vi "Raster_2DOutput_wCounter_82_EXP_ODMR pulsing.vi"(2 "Save File path":path, 3 "Save?":bool=TRUE, 6 "error in":errorcluster, 7 "Update Rate (Hz)":dbl=100.0, 8 "Y Parameters":T1={"Number of Y Steps"=200, "Max Y (V)"=1.0, "Min Y (V)"=-1.0}, 9 "X Parameters":T2={"Number of X Steps"=200, "Max X (V)"=1.0, "Min X (V)"=-1.0}) -> (0 "error out":errorcluster, 1 "Intensity Graph":dbl[][](graph))   [LabVIEW 2012]
uses:
  <vilib>/DAQmx/write.llb/DAQmx Write (Analog 2D DBL NChan NSamp).vi
  <vilib>/DAQmx/read.llb/DAQmx Read (Counter 1D U32 1Chan NSamp).vi
  <vilib>/DAQmx/create/channels.llb/DAQmx Create Channel (CI-Count Edges).vi
  <vilib>/DAQmx/create/channels.llb/DAQmx Create Channel (AO-Voltage-Basic).vi
  <vilib>/DAQmx/configure/timing.llb/DAQmx Timing (Sample Clock).vi
  <vilib>/DAQmx/miscellaneous.llb/DAQmx Fill In Error Info.vi
  <resource>/objmgr/daqmx.rc
panel:
  out "Intensity Graph 3":dbl[][](graph)
  out "Intensity Graph 2":dbl[][](graph)
  out "TotalSampPerChanAcquired 2":dbl=5601.0
  out "TotalSampPerChanAcquired":dbl=5601.0
  out "Output:":dbl[][](graph)
  in  "stop":bool
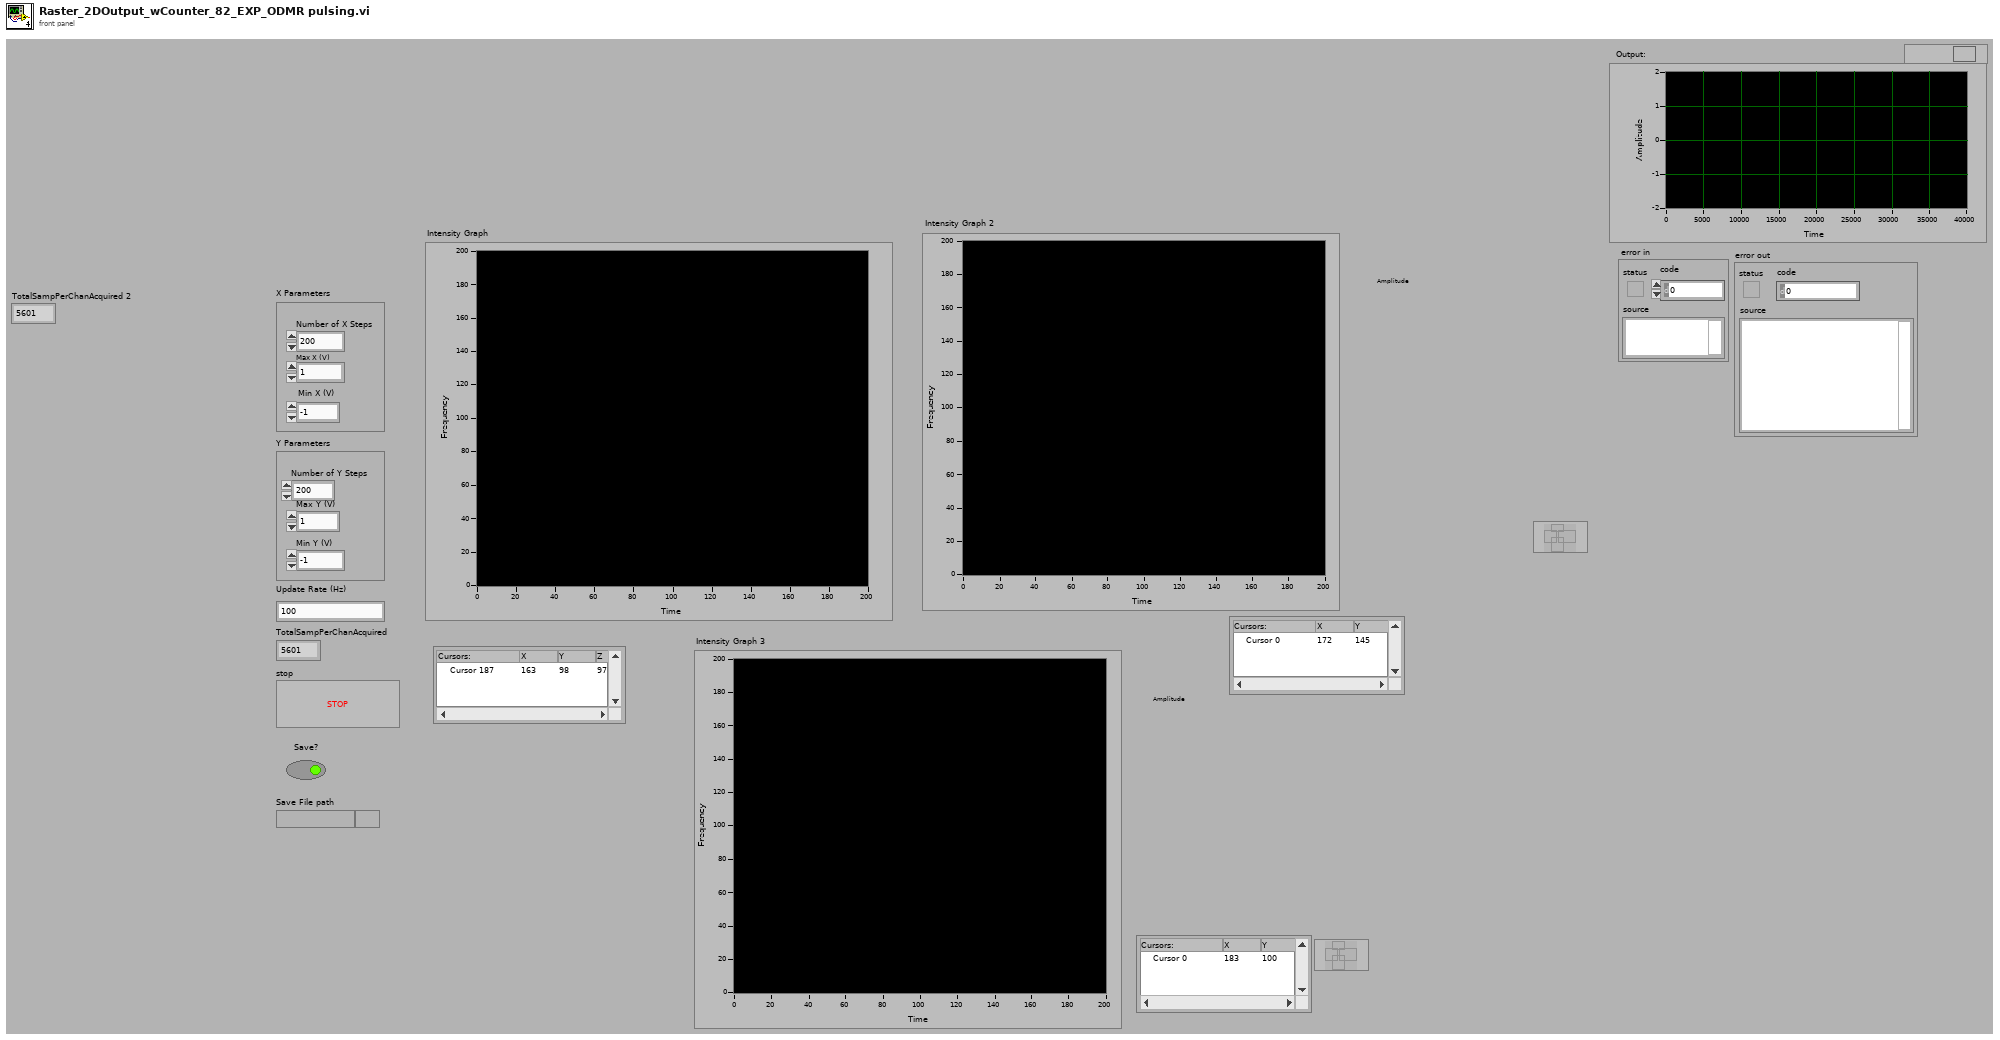
[diagram p1: front panel]
types:
  T1 = cluster{"Number of Y Steps":i32, "Max Y (V)":dbl, "Min Y (V)":dbl}
  T2 = cluster{"Number of X Steps":i32, "Max X (V)":dbl, "Min X (V)":dbl}
  T3 = typedef "imagedata.ctl" = cluster{"image type":i32, "image depth":i32, "image":u8[], "mask":u8[], "colors":u32[], "Rectangle":cluster{"left":i16, "top":i16, "right":i16, "bottom":i16}}
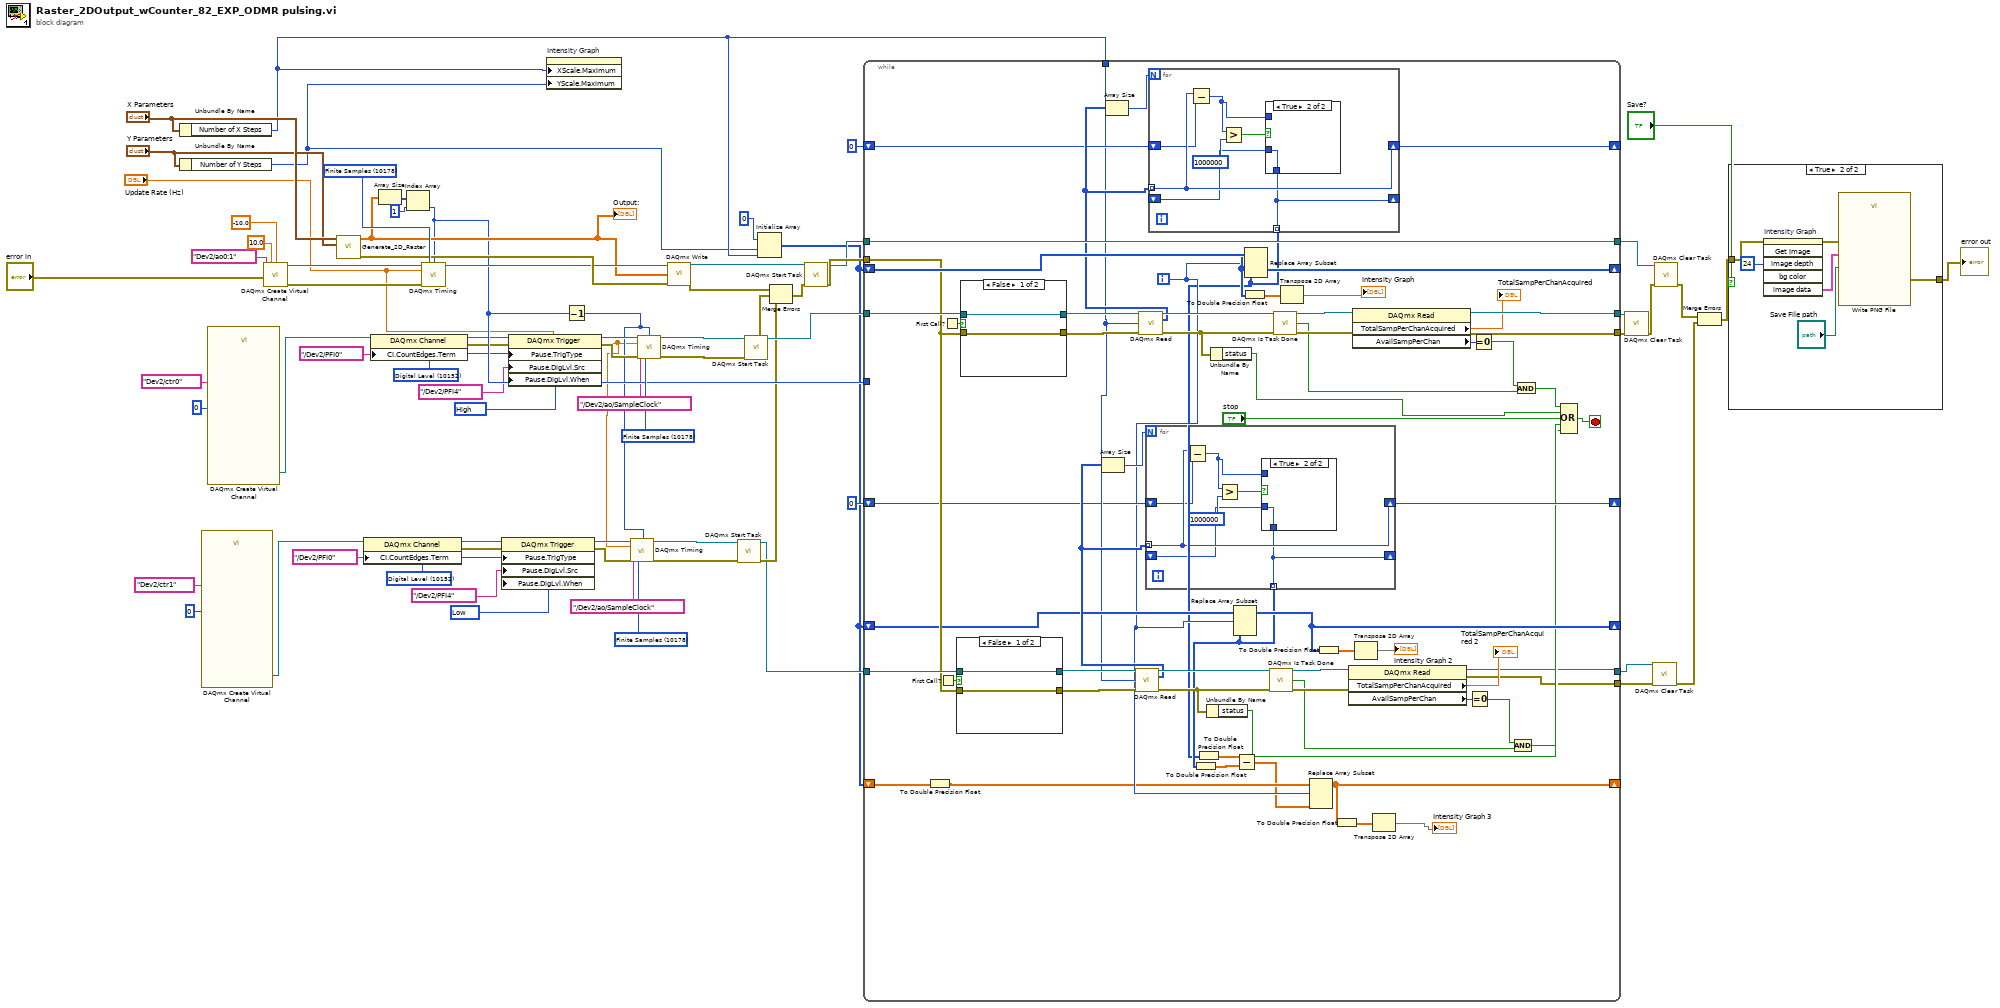
[diagram p0: block diagram]
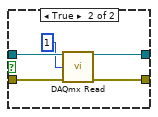
[diagram p4: hidden frame]
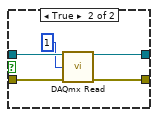
[diagram p6: hidden frame]
diagram:
  w12 = 10214 items=["High"=10192, "Low"=10214] ("Pause.DigLvl.When")
  w14 = 10152 items=["Analog Level"=10101, "Analog Window"=10103, "Digital Level"=10152, "Digital Pattern"=10398, "None"=10230] ("Pause.TrigType")
  w25 = 10178 items=["Finite Samples"=10178, "Continuous Samples"=10123, "Hardware Timed Single Point"=12522] ("sample mode")
  w27 = 10192 items=["High"=10192, "Low"=10214] ("Pause.DigLvl.When")
  w29 = 10152 items=["Analog Level"=10101, "Analog Window"=10103, "Digital Level"=10152, "Digital Pattern"=10398, "None"=10230] ("Pause.TrigType")
  w64 = 10178 items=["Finite Samples"=10178, "Continuous Samples"=10123, "Hardware Timed Single Point"=12522] ("sample mode")
  w65 = 10178 items=["Finite Samples"=10178, "Continuous Samples"=10123, "Hardware Timed Single Point"=12522] ("sample mode")
  n1 = Unbundle By Name("X Parameters") -> ("Number of X Steps"=w34:i32)
  n2 = Unbundle By Name("Y Parameters") -> ("Number of Y Steps"=w33:i32)
  n3 = call-poly <vilib>:"DAQmx Create Virtual Channel.vi"("initial count"=u32 0, "counter"=tag "Dev2/ctr1") -> ("task out"=w23:refnum<k21>)  [unwired: 6 in, 7 out]
  n4 = call-poly <vilib>:"DAQmx Create Virtual Channel.vi"("initial count"=u32 0, "counter"=tag "Dev2/ctr0") -> ("task out"=w42:refnum<k21>)  [unwired: 6 in, 7 out]
  n5 = call-poly <vilib>:"DAQmx Create Virtual Channel.vi"("maximum value"=10.0, "minimum value"=-10.0, "physical channels"=tag "Dev2/ao0:1", "error in"="error in") -> ("task out"=w73:refnum<k21>, "error out"=w72:errorcluster)  [unwired: 5 in, 5 out]
  n6 = call "Generate_2D_Raster.vi"("Y Parameters"="Y Parameters", "X Parameters"="X Parameters") -> ("error IO"=w56:errorcluster, "Array"=w51:dbl[][])  [unwired: 1 in, 7 out]
  "Output:" <- w51
  n7 = property class="DAQmx Channel"(reference=w23, "CI.CountEdges.Term"=tag "/Dev2/PFI0") -> (reference out=w22:refnum<k21>, error out=w16:errorcluster)  [unwired: 1 in]
  n8 = property class="DAQmx Channel"(reference=w42, "CI.CountEdges.Term"=tag "/Dev2/PFI0") -> (reference out=w41:refnum<k21>, error out=w31:errorcluster)  [unwired: 1 in]
  n9 = Array Size(array=w51) -> (size(s)=w50:i32[])
  n10 = Index Array(array=w50, index=1) -> (element=w48:i32)
  n11 = call-poly <vilib>:"DAQmx Timing.vi"("task/channels in"=w73, "sample mode"=w65, "samples per channel"=w48, "rate"="Update Rate (Hz)", "error in"=w72) -> ("task out"=w52:refnum<k21>)  [unwired: 2 in, 8 out]
  n12 = property class="DAQmx Trigger"(reference=w22, error in=w16, "Pause.TrigType"=w14, "Pause.DigLvl.Src"=tag "/Dev2/PFI4", "Pause.DigLvl.When"=w12) -> (reference out=w17:refnum<k21>, error out=w15:errorcluster)
  n13 = property class="DAQmx Trigger"(reference=w41, error in=w31, "Pause.TrigType"=w29, "Pause.DigLvl.Src"=tag "/Dev2/PFI4", "Pause.DigLvl.When"=w27) -> (reference out=w32:refnum<k21>, error out=w30:errorcluster)
  n14 = property on="Intensity Graph" class="IntGraph (strict)"("XScale.Maximum"=w34, "YScale.Maximum"=w33) -> ()  [unwired: 2 in, 2 out]
  n15 = Decrement(x=w48) -> (x-1=w11:i32)
  n16 = call-poly <vilib>:"DAQmx Timing.vi"("task/channels in"=w17, "sample mode"=w25, "samples per channel"=w11, "rate"="Update Rate (Hz)", "source"=tag "/Dev2/ao/SampleClock", "error in"=w15) -> ("task out"=w26:refnum<k21>, "error out"=w18:errorcluster)  [unwired: 1 in, 7 out]
  n17 = call-poly <vilib>:"DAQmx Timing.vi"("task/channels in"=w32, "sample mode"=w64, "samples per channel"=w11, "rate"="Update Rate (Hz)", "source"=tag "/Dev2/ao/SampleClock", "error in"=w30) -> ("task out"=w70:refnum<k21>, "error out"=w35:errorcluster)  [unwired: 1 in, 7 out]
  n18 = call-poly <vilib>:"DAQmx Write.vi"("task/channels in"=w52, "data"=w51, "error in"=w56) -> ("task out"=w69:refnum<k21>, "error out"=w58:errorcluster)  [unwired: 1 in, 10 out]
  n19 = call <vilib>:"DAQmx Start Task.vi"("task/channels in"=w26, "error in"=w18) -> ("task out"=w9:refnum<k21>, "error out"=w10:errorcluster)  [unwired: 12 out]
  n20 = call <vilib>:"DAQmx Start Task.vi"("task/channels in"=w70, "error in"=w35) -> ("task out"=w66:refnum<k21>, "error out"=w57:errorcluster)  [unwired: 12 out]
  n21 = Initialize Array(u32 0, w33, w34) -> (w2:u32[][])
  n22 = Merge Errors(w58, w57, w10) -> (w59:errorcluster)
  n23 = call <vilib>:"DAQmx Start Task.vi"("task/channels in"=w69, "error in"=w59) -> ("task out"=w67:refnum<k21>, "error out"=w68:errorcluster)  [unwired: 12 out]
  n24 = while {
    tunnel: w67 -> [w130]
    tunnel: w68 -> [w94]
    tunnel: w66 -> [w136]
    tunnel: [w130] -> w63
    tunnel: w34 -> [w91]
    shift-right: [w131] -> _
    shift-left: w2 -> [w132]
    tunnel: w48 -> [_]
    tunnel: [w126] -> w47
    tunnel: [w127] -> w46
    shift-right: [w113] -> _
    shift-left: u32 0 ("Numeric") -> [w112]
    tunnel: w9 -> [w95]
    shift-right: [w92] -> _
    shift-left: w2 -> [w93]
    shift-right: [w89] -> _
    shift-left: u32 0 ("Numeric") -> [w90]
    tunnel: [w86] -> w7
    tunnel: [w85] -> w6
    shift-right: [w82] -> _
    shift-left: w2 -> [w79]
    i -> [w83]
    stop <- w137 stop-if-true
    n25 = To Double Precision Float(number=w79) -> (double precision float=w78:dbl[][])
    n26 = First Call?() -> (First Call?: T/F=w108:bool)
    n27 = First Call?() -> (First Call?: T/F=w133:bool)
    n28 = case shown="False" w108 {
      tunnel: w95 -> [w148 w153]
      tunnel: [w148 w152] -> w110
      tunnel: [w147 w151] -> w109
      tunnel: w94 -> [w147 w150]
      frame False {
      }
      frame True {
        n29 = call-poly <vilib>:"DAQmx Read.vi"("task/channels in"=w153, "number of samples per channel"=1, "error in"=w150) -> ("task out"=w152:refnum<k21>, "error out"=w151:errorcluster)  [unwired: 11 out]
      }
    }
    n30 = case shown="False" w133 {
      tunnel: w136 -> [w164 w169]
      tunnel: [w164 w168] -> w135
      tunnel: [w163 w167] -> w134
      tunnel: w94 -> [w163 w166]
      frame False {
      }
      frame True {
        n31 = call-poly <vilib>:"DAQmx Read.vi"("task/channels in"=w169, "number of samples per channel"=1, "error in"=w166) -> ("task out"=w168:refnum<k21>, "error out"=w167:errorcluster)  [unwired: 11 out]
      }
    }
    n32 = call-poly <vilib>:"DAQmx Read.vi"("task/channels in"=w110, "number of samples per channel"=w91, "error in"=w109) -> ("task out"=w106:refnum<k21>, "data"=w97:u32[], "error out"=w99:errorcluster)  [unwired: 1 in, 9 out]
    n33 = Array Size(array=w97) -> (size(s)=w98:i32)
    n34 = call-poly <vilib>:"DAQmx Read.vi"("task/channels in"=w135, "number of samples per channel"=w91, "error in"=w134) -> ("task out"=w128:refnum<k21>, "data"=w114:u32[], "error out"=w119:errorcluster)  [unwired: 1 in, 9 out]
    n35 = Array Size(array=w114) -> (size(s)=w115:i32)
    n36 = for {
      N: w98 -> [_]
      tunnel: w97 -> [w144] mode=indexing
      shift-right: [w144] -> w89
      shift-left: w90 -> [w143]
      tunnel: [w139] -> w81 mode=indexing
      shift-right: [w139] -> _
      shift-left: _ -> [w138]
      n37 = Subtract(x=w144, y=w143) -> (x-y=w140:u32)
      n38 = Greater?(x=w140, y=u32 1000000) -> (0:w141:bool)
      n39 = case shown="True" w141 {
        tunnel: w140 -> [w145 _]
        tunnel: [w145 w146] -> w139
        tunnel: w138 -> [_ w146]
        frame False {
        }
        frame True {
        }
      }
    }
    n40 = for {
      N: w115 -> [_]
      tunnel: w114 -> [w160] mode=indexing
      shift-right: [w160] -> w113
      shift-left: w112 -> [w159]
      tunnel: [w155] -> w80 mode=indexing
      shift-right: [w155] -> _
      shift-left: _ -> [w154]
      n41 = Subtract(x=w160, y=w159) -> (x-y=w156:u32)
      n42 = Greater?(x=w156, y=u32 1000000) -> (0:w157:bool)
      n43 = case shown="True" w157 {
        tunnel: w156 -> [w161 _]
        tunnel: [w161 w162] -> w155
        tunnel: w154 -> [_ w162]
        frame False {
        }
        frame True {
        }
      }
    }
    n44 = To Double Precision Float(number=w81) -> (double precision float=w77:dbl[])
    n45 = To Double Precision Float(number=w80) -> (double precision float=w76:dbl[])
    n46 = Unbundle By Name(w99) -> ("status"=w88:bool)
    n47 = Unbundle By Name(w119) -> ("status"=w117:bool)
    n48 = Replace Array Subset(array=w93, new element=w81, index (row)=w83) -> (w92:u32[][])  [unwired: 1 in]
    n49 = Subtract(x=w76, y=w77) -> (x-y=w75:dbl[])
    n50 = Replace Array Subset(array=w132, new element=w80, index (row)=w83) -> (w131:u32[][])  [unwired: 1 in]
    n51 = To Double Precision Float(number=w131) -> (double precision float=w129:dbl[][])
    n52 = call <vilib>:"DAQmx Is Task Done.vi"("task/channels in"=w106, "error in"=w99) -> ("task out"=w105:refnum<k21>, "task done?"=w102:bool, "error out"=w104:errorcluster)  [unwired: 11 out]
    n53 = call <vilib>:"DAQmx Is Task Done.vi"("task/channels in"=w128, "error in"=w119) -> ("task out"=w125:refnum<k21>, "task done?"=w122:bool, "error out"=w124:errorcluster)  [unwired: 11 out]
    n54 = Transpose 2D Array(2D array=w129) -> (transposed array=→"Intensity Graph":dbl[][])
    n55 = Replace Array Subset(array=w78, new element=w75, index (row)=w83) -> (w82:dbl[][])  [unwired: 1 in]
    n56 = To Double Precision Float(number=w92) -> (double precision float=w107:dbl[][])
    n57 = To Double Precision Float(number=w82) -> (double precision float=w84:dbl[][])
    n58 = property class="DAQmx Read"(reference=w105, error in=w104) -> (reference out=w86:refnum<k21>, error out=w85:errorcluster, "TotalSampPerChanAcquired"=→"TotalSampPerChanAcquired 2":dbl, "AvailSampPerChan"=w101:u32)
    n59 = property class="DAQmx Read"(reference=w125, error in=w124) -> (reference out=w127:refnum<k21>, error out=w126:errorcluster, "TotalSampPerChanAcquired"=→"TotalSampPerChanAcquired":dbl, "AvailSampPerChan"=w121:u32)
    n60 = Transpose 2D Array(2D array=w107) -> (transposed array=→"Intensity Graph 2":dbl[][])
    n61 = Transpose 2D Array(2D array=w84) -> (transposed array=→"Intensity Graph 3":dbl[][])
    n62 = Equal To 0?(x=w101) -> (x = 0?=w100:bool)
    n63 = Equal To 0?(x=w121) -> (x = 0?=w120:bool)
    n64 = And(x=w100, y=w102) -> (x .and. y?=w87:bool)
    n65 = And(x=w120, y=w122) -> (x .and. y?=w116:bool)
    n66 = Compound Arithmetic op=OR(w116, w117, "stop", w88, w87) -> (w137:bool)
  }
  n67 = call <vilib>:"DAQmx Clear Task.vi"("task in"=w46, "error in"=w47) -> ("error out"=w60:errorcluster)  [unwired: 13 out]
  n68 = call <vilib>:"DAQmx Clear Task.vi"("task in"=w7, "error in"=w6) -> ("error out"=w3:errorcluster)  [unwired: 13 out]
  n69 = call <vilib>:"DAQmx Clear Task.vi"("task in"=w63, "error in"=w60) -> ("error out"=w5:errorcluster)  [unwired: 13 out]
  n70 = Merge Errors(w5, w3) -> (w4:errorcluster)
  n71 = case shown="True" "Save?" {
    tunnel: w4 -> [w170 w174]
    tunnel: [w170 w176] -> w45
    frame False {
    }
    frame True {
      n72 = invoke on="Intensity Graph" class="IntGraph (strict)" method="Get Image"(error in=w174, "image depth"=24 ("Image Depth")) -> (error out=w173:errorcluster, "image data"=w172:T3)  [unwired: 4 in, 4 out]
      n73 = call <vilib>:"Write PNG File.vi"("error in (no error)"=w173, "image data"=w172, "path to PNG file"="Save File path") -> ("error out"=w176:errorcluster)  [unwired: 7 in, 1 out]
    }
  }
  "error out" <- w45
